vi "LTbridgeOnChipCalibration.vi"(4 "C ref, pF":dbl, 6 "V exc sample":dbl, 7 "SR830 1 addr":u8, 9 "pm":dbl, 10 "V exc ref (SR830_2)":dbl, 11 "SR830 2 addr":u8) -> (0 "Array":cluster{dbl[], "Best Linear Fit":dbl[]}[](array[cluster]), 1 "Numeric 2":dbl, 2 "Numeric":dbl, 3 "R-square":dbl)   [LabVIEW 2017]
uses:
  <vilib>/Analysis/1siggen.llb/Ramp Pattern by Samples.vi
  <vilib>/Analysis/NI_AALPro.lvlib
  <vilib>/Analysis/NI_AALBase.lvlib
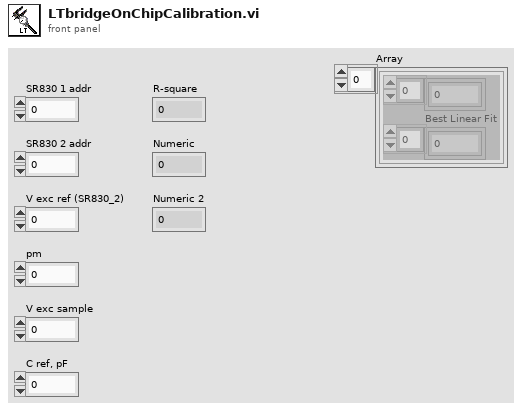
[diagram p1: front panel]
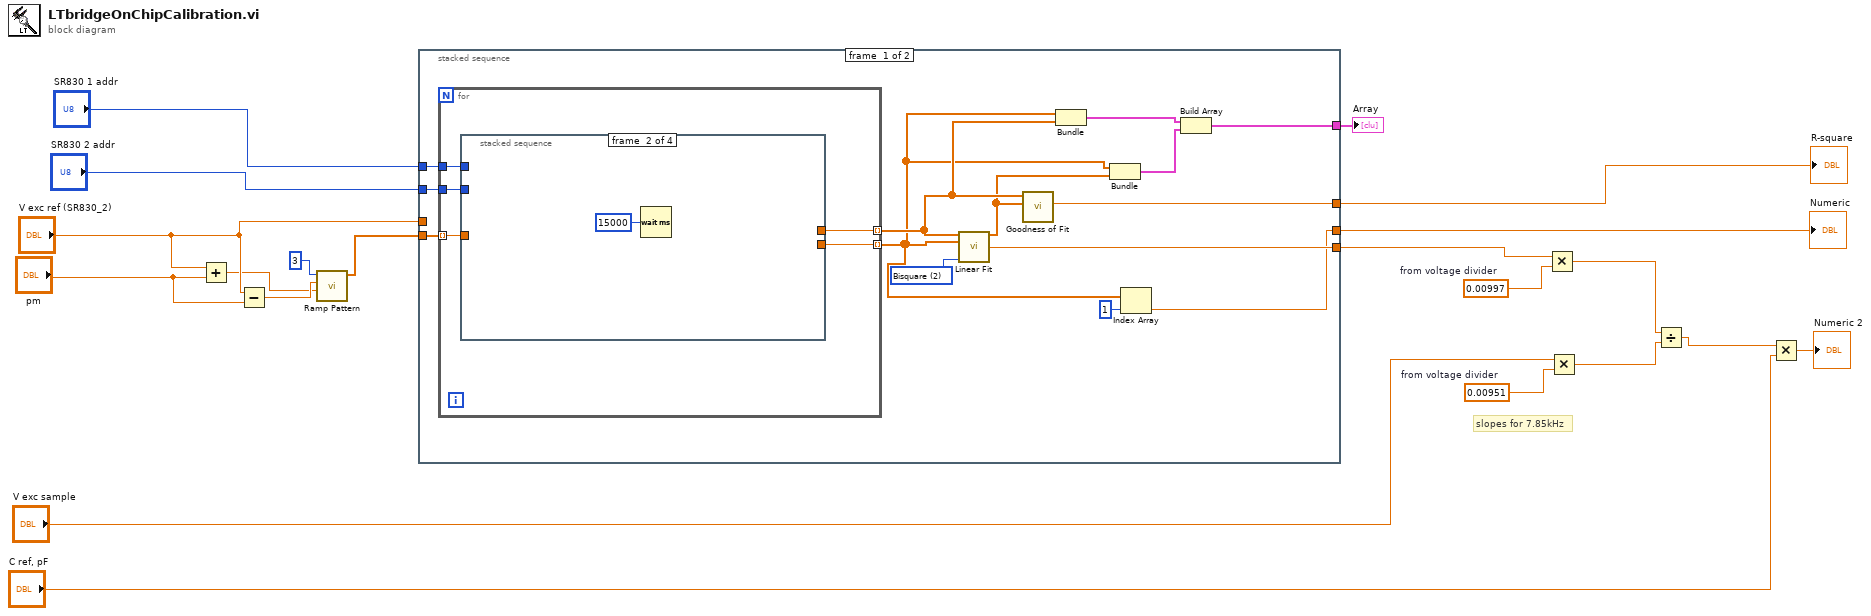
[diagram p0: block diagram]
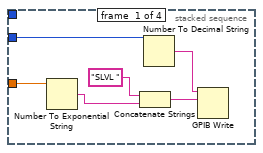
[diagram p2: hidden frame]
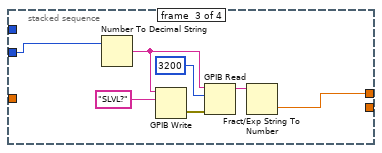
[diagram p3: hidden frame]
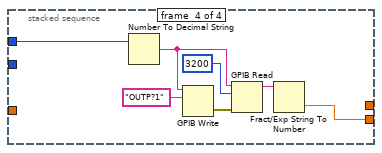
[diagram p4: hidden frame]
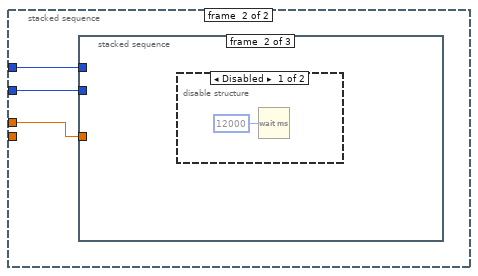
[diagram p5: hidden frame]
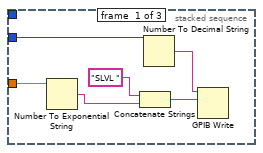
[diagram p6: hidden frame]
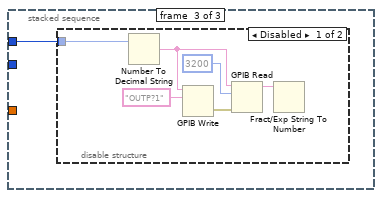
[diagram p8: hidden frame]
diagram:
  w13 = 0.00951  # from voltage divider
  w12 = 0.00997  # from voltage divider
  # "slopes for 7.85kHz"
  n1 = Add(x="V exc ref (SR830_2)", y="pm") -> (x+y=w6:dbl)
  n2 = Subtract(x="V exc ref (SR830_2)", y="pm") -> (x-y=w7:dbl)
  n3 = call-poly <vilib>:"Ramp Pattern.vi"("start"=w6, "end"=w7, "samples"=3) -> ("Ramp Pattern"=w8:dbl[])  [unwired: 7 in, 1 out]
  n4 = stacked-sequence {
    tunnel: "SR830 2 addr" -> [w34 w62]
    tunnel: "SR830 1 addr" -> [w33 w63]
    tunnel: w8 -> [w32 _]
    tunnel: "V exc ref (SR830_2)" -> [_ w61]
    tunnel: [w21 _] -> w20
    tunnel: [w30 _] -> w11
    tunnel: [w29 _] -> w10
    tunnel: [w24 _] -> w1
    frame #0 {
      w31 = u16 2 items=["Least Square", "Least Absolute Residual", "Bisquare"] ("method")
      n5 = for {
        tunnel: w34 -> [w39]
        tunnel: w33 -> [w38]
        tunnel: w32 -> [w37] mode=indexing
        tunnel: [w35] -> w28 mode=indexing
        tunnel: [w36] -> w23 mode=indexing
        n6 = stacked-sequence {
          tunnel: w39 -> [w44 _ w48 _]
          tunnel: w37 -> [w40 _ _ _]
          tunnel: w38 -> [_ _ _ w55]
          tunnel: [_ _ _ w54] -> w36
          tunnel: [_ _ w47 _] -> w35
          frame #0 {
            n7 = Number To Exponential String(number=w40) -> (E-format string=w43:string)  [unwired: 3 in]
            n8 = Concatenate Strings("SLVL ", w43) -> (w41:string)
            n9 = Number To Decimal String(number=w44) -> (decimal integer string=w45:string)  [unwired: 1 in]
            n10 = GPIB Write(0:w45, 1:w41) -> ()  [unwired: 3 in, 2 out]
          }
          frame #1 {
            n11 = Wait (ms)(milliseconds to wait=u32 15000) -> ()  [unwired: 1 out]
          }
          frame #2 {
            n12 = Number To Decimal String(number=w48) -> (decimal integer string=w49:string)  [unwired: 1 in]
            n13 = GPIB Write(0:w49, 1:"SLVL?") -> (6:w53:errorcluster)  [unwired: 3 in, 1 out]
            n14 = GPIB Read(0:w49, 1:3200, 3:w53) -> (5:w51:string)  [unwired: 2 in, 2 out]
            n15 = Fract/Exp String To Number(string=w51) -> (number=w47:dbl)  [unwired: 3 in, 1 out]
          }
          frame #3 {
            n16 = Number To Decimal String(number=w55) -> (decimal integer string=w56:string)  [unwired: 1 in]
            n17 = GPIB Write(0:w56, 1:"OUTP?1") -> (6:w60:errorcluster)  [unwired: 3 in, 1 out]
            n18 = GPIB Read(0:w56, 1:3200, 3:w60) -> (5:w58:string)  [unwired: 2 in, 2 out]
            n19 = Fract/Exp String To Number(string=w58) -> (number=w54:dbl)  [unwired: 3 in, 1 out]
          }
        }
      }
      n20 = call <vilib>:"Linear Fit.vi"("Y"=w28, "X"=w23, "method"=w31) -> ("Best Linear Fit"=w27:dbl[], "intercept"=w30:dbl)  [unwired: 8 in, 3 out]
      n21 = call <vilib>:"Goodness of Fit.vi"("Best Fit"=w27, "Y"=w28) -> ("R-square"=w29:dbl)  [unwired: 6 in, 3 out]
      n22 = Bundle(w23, w28) -> (w26:cluster{dbl[], dbl[]})  [unwired: 1 in]
      n23 = Bundle(w23, "Best Linear Fit"=w27) -> (w25:cluster{dbl[], "Best Linear Fit":dbl[]})  [unwired: 1 in]
      n24 = Index Array(array=w23, index=1) -> (element=w21:dbl)
      n25 = Build Array(w26, w25) -> (w24:cluster{dbl[], "Best Linear Fit":dbl[]}[])
    }
    frame #1 {
      n26 = stacked-sequence {
        tunnel: w62 -> [w68 _ _]
        tunnel: w61 -> [w64 _ _]
        tunnel: w63 -> [_ _ w71]
        frame #0 {
          n27 = Number To Exponential String(number=w64) -> (E-format string=w67:string)  [unwired: 3 in]
          n28 = Concatenate Strings("SLVL ", w67) -> (w65:string)
          n29 = Number To Decimal String(number=w68) -> (decimal integer string=w69:string)  [unwired: 1 in]
          n30 = GPIB Write(0:w69, 1:w65) -> ()  [unwired: 3 in, 2 out]
        }
        frame #1 {
          n31 = disable-structure shown="Disabled" {
            frame Disabled {
              n32 = Wait (ms)(milliseconds to wait=u32 12000) -> ()  [unwired: 1 out]
            }
            frame Enabled {
            }
          }
        }
        frame #2 {
          n33 = disable-structure shown="Disabled" {
            disable-tunnel: w71 -> [w72 _]
            frame Disabled {
              n34 = Number To Decimal String(number=w72) -> (decimal integer string=w73:string)  [unwired: 1 in]
              n35 = GPIB Write(0:w73, 1:"OUTP?1") -> (6:w77:errorcluster)  [unwired: 3 in, 1 out]
              n36 = GPIB Read(0:w73, 1:3200, 3:w77) -> (5:w75:string)  [unwired: 2 in, 2 out]
              n37 = Fract/Exp String To Number(string=w75) -> ()  [unwired: 3 in, 2 out]
            }
            frame Enabled {
            }
          }
        }
      }
    }
  }
  "Numeric" <- w20
  "R-square" <- w10
  "Array" <- w1
  n38 = Multiply(x=w11, y=w12) -> (x*y=w15:dbl)
  n39 = Multiply(x="V exc sample", y=w13) -> (x*y=w16:dbl)
  n40 = Divide(x=w15, y=w16) -> (x/y=w17:dbl)
  n41 = Multiply(x=w17, y="C ref, pF") -> (x*y=→"Numeric 2":dbl)
